vi "Password Authentication.vi"(8 "Error In":errorcluster, 10 "Password":string, 11 "Username":string="cfield") -> (0 "Error Out":errorcluster)   [LabVIEW 2017, in "Tests.lvlib" / "Session.lvlib"]
uses:
  Session.lvlib
  <vilib>/addons/_JKI Toolkits/Caraya/classes/Test/Test.lvclass
  src/Toolkit/Toolkit.lvlib
  src/Toolkit/API/Session/Session.lvclass
  <vilib>/addons/_JKI Toolkits/Caraya/classes/Assert/Assert.lvclass
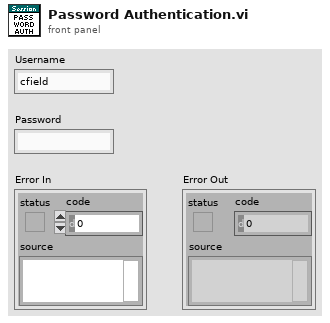
[diagram p1: front panel]
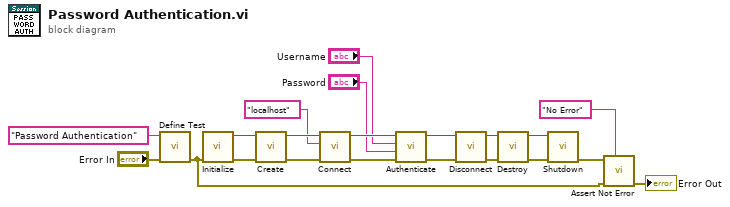
[diagram p0: block diagram]
diagram:
  n1 = call <vilib>:"Define Test.vi"("error in (no error)"="Error In", "Label (VI Title)"="Password Authentication") -> ("error out"=w13:errorcluster)  [unwired: 9 in]
  n2 = call "Initialize.vi"("Error In"=w13) -> ("Error Out"=w19:errorcluster, "lv-libssh2 Shared Library Out"=w18:path)  [unwired: 9 in]
  n3 = call "Create.vi"("Error In"=w19, "lv-libssh2 Shared Library"=w18) -> ("Error Out"=w10:errorcluster, "Sesssion"=w11:refnum<class "Session.lvclass">)  [unwired: 8 in]
  n4 = call "Connect.vi"("Error In"=w10, "Address"="localhost", "Session In"=w11) -> ("Error Out"=w5:errorcluster, "Sesssion Out"=w6:refnum<class "Session.lvclass">)  [unwired: 7 in]
  n5 = call-poly "Authenticate.vi"("Error In"=w5, "Password"="Password", "Username"="Username", "Session In"=w6) -> ("Error Out"=w3:errorcluster, "Sesssion Out"=w4:refnum<class "Session.lvclass">)  [unwired: 6 in]
  n6 = call "Disconnect.vi"("Error In"=w3, "Session In"=w4) -> ("Error Out"=w7:errorcluster, "Sesssion Out"=w8:refnum<class "Session.lvclass">)  [unwired: 8 in]
  n7 = call "Destroy.vi"("Error In"=w7, "Session"=w8) -> ("Error Out"=w16:errorcluster, "lv-libssh2 Shared Library"=w17:path)  [unwired: 8 in]
  n8 = call "Shutdown.vi"("Error In"=w16, "lv-libssh2 Shared Library"=w17) -> ("Error Out"=w15:errorcluster)  [unwired: 9 in]
  n9 = call <vilib>:"Assert Not Error.vi"("Label"="No Error", "error in (no error)"=w13, "Not Error?"=w15) -> ("error out"=→"Error Out":errorcluster)  [unwired: 8 in]
